vi "pruebausuario.vi"() -> ()   [LabVIEW 2018]
uses:
  Tabcontrol.ctl
panel:
  out "element":string
  out "Tab Control 2":enum32{"Login", "Usuarios", "Admin"}(tab)
  in  "Usuario 2":string
  in  "Contraseña 4":string
  in  "ingresar":bool
  in  "Contraseña U.I":string
  in  "Usuario a Ingresar":string
  in  "OK Button":bool
  in  "eliminar 2":bool
  out "array":string[][](array[string])
  out "result string":string
  out "Boolean":bool
  out "Contraseña 3":string
  in  "stop":bool
  out "appended path":path
  out "before substring":string
  out "match substring":string
  out "after substring":string
  out "text":string
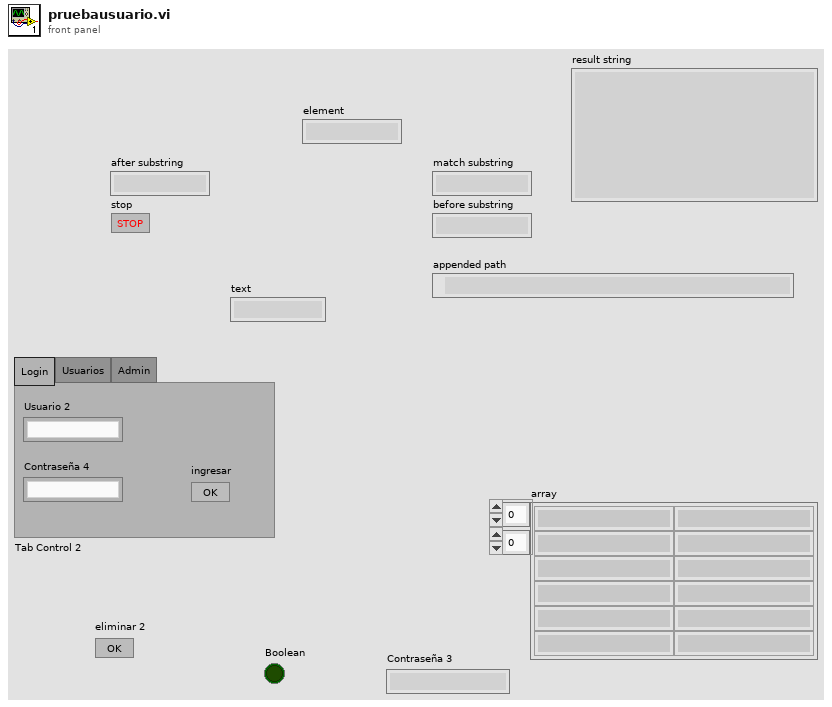
[diagram p1: front panel]
types:
  T1 = typedef "Tabcontrol.ctl" = enum16{"Login", "Usuarios", "Admin"}
  T2 = enum16{"open", "replace", "create", "open or create", "replace or create", "replace or create with confirmation"}
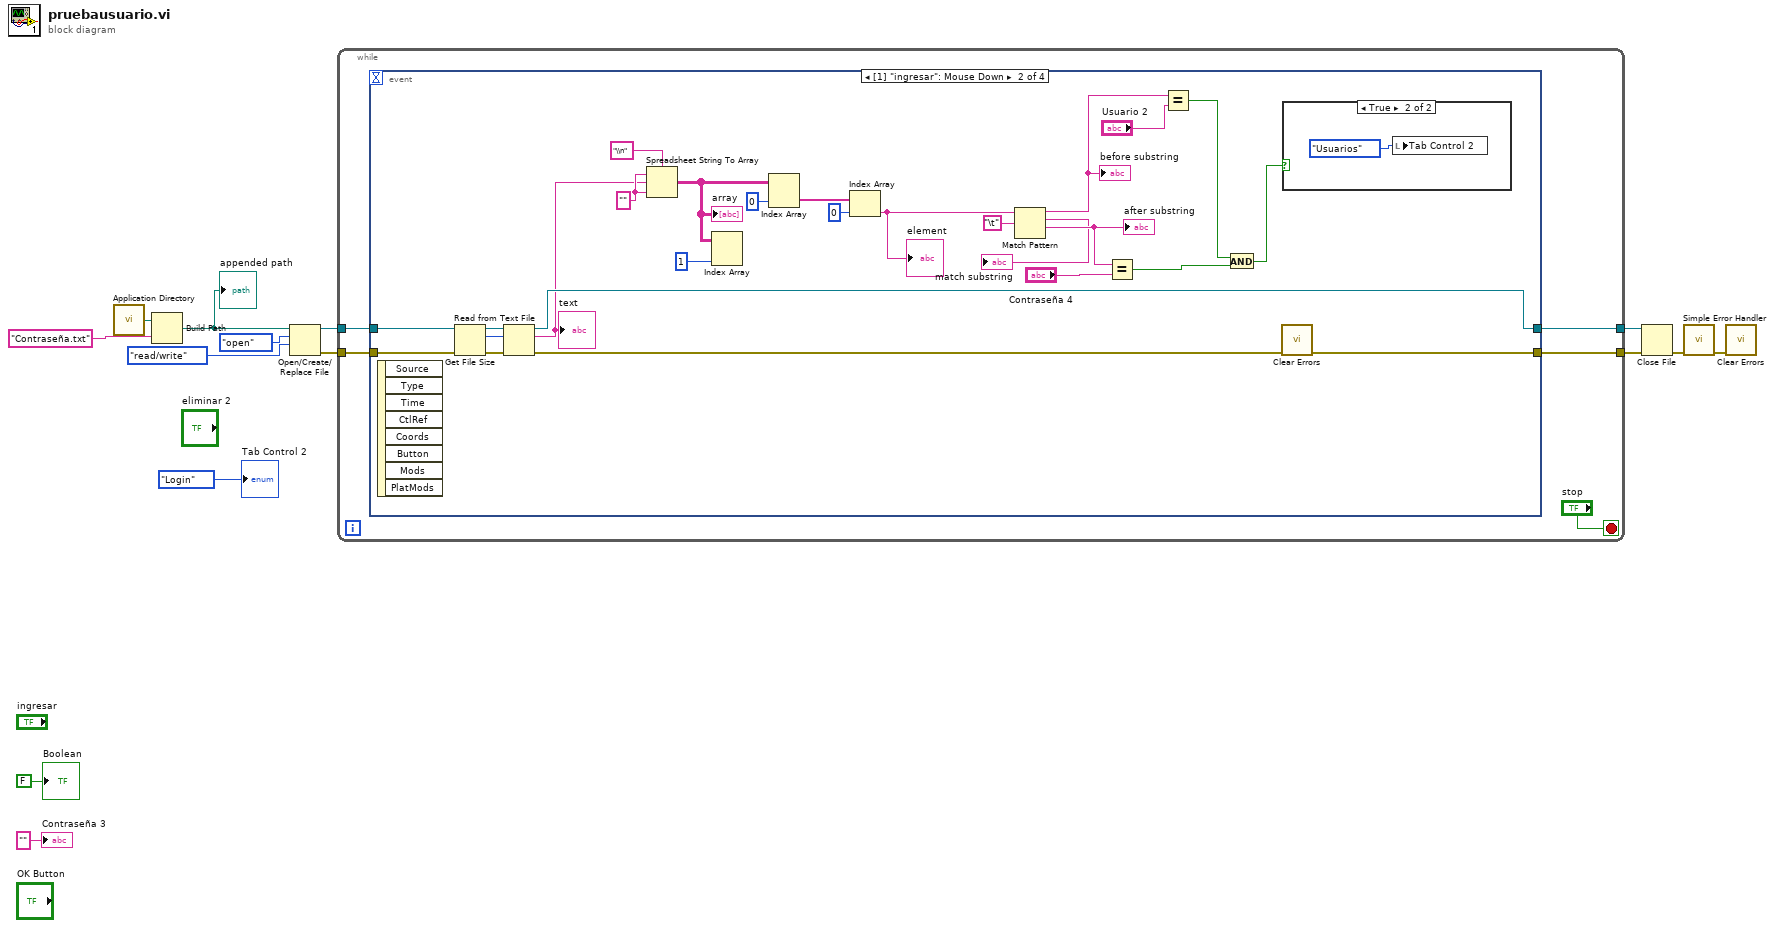
[diagram p0: block diagram]
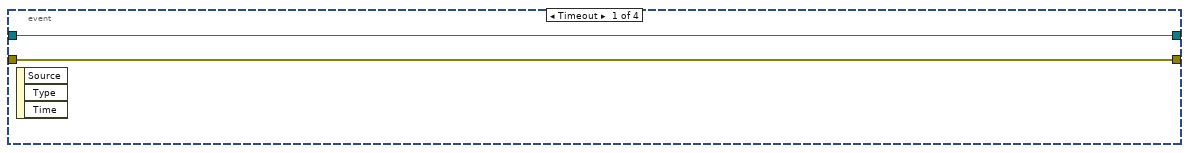
[diagram p2: hidden frame]
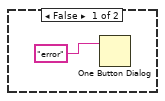
[diagram p3: hidden frame]
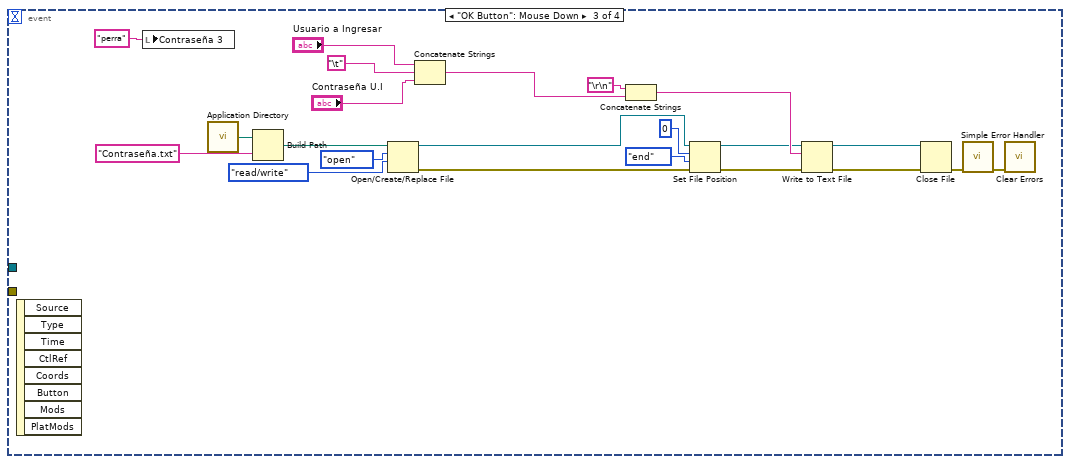
[diagram p4: hidden frame]
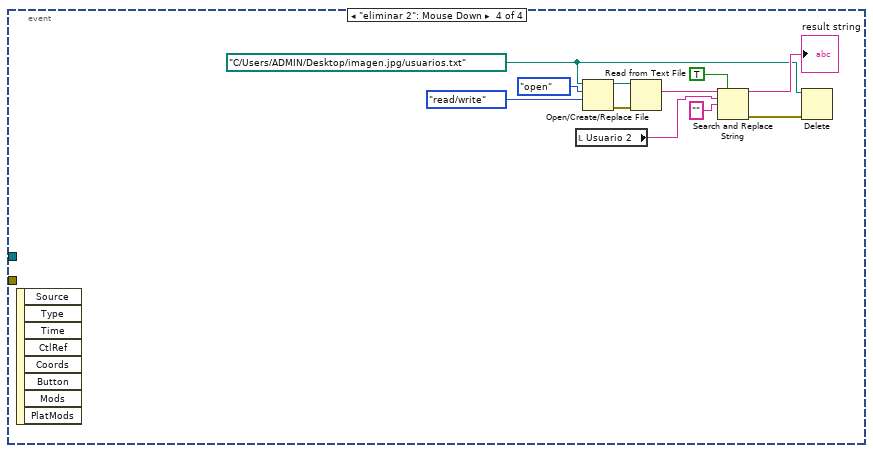
[diagram p5: hidden frame]
diagram:
  n1 = call <vilib>:"Application Directory.vi"() -> ("Application Directory"=w14:path)
  n2 = Build Path(base path=w14, name or relative path="Contraseña.txt") -> (appended path=w12:path)
  "appended path" <- w12
  n3 = Open/Create/Replace File(file path (use dialog)=w12, operation (0:open)=T2."open", access (0:read/write)=enum16{"read/write", "read-only", "write-only"}."read/write") -> (refnum out=w10:refnum<file>, error out=w11:errorcluster)  [unwired: 3 in, 1 out]
  n4 = while {
    tunnel: w11 -> [w19]
    tunnel: w10 -> [w18]
    tunnel: [w17] -> w9
    tunnel: [w16] -> w8
    stop <- "stop" stop-if-true
    n5 = event shown="[1] \"ingresar\": Mouse Down" {
      selector: _ -> [_ _ _ _]
      dyn-events: _ -> [_ _ _ _]
      timeout: _ -> [_ _ _ _]
      tunnel: w19 -> [w20 w37 _ _]
      tunnel: w18 -> [w21 w38 _ _]
      tunnel: [w20 w33 _ _] -> w17
      tunnel: [w21 w40 _ _] -> w16
      event Timeout {
        n6 = event-data() -> ()  [unwired: 1 in, 3 out]
      }
      event "ingresar": Mouse Down {
        w32 = "" ("format string")
        n7 = event-data() -> ()  [unwired: 1 in, 8 out]
        n8 = Get File Size(file=w38, error in=w37) -> (refnum out=w35:refnum<file>, size (in bytes)=w34:i64, 0:w36:errorcluster)
        n9 = Read from Text File(file (use dialog)=w35, count=w34, error in=w36) -> (refnum out=w40:refnum<file>, text=w31:string, error out=w41:errorcluster)  [unwired: 1 in, 1 out]
        "text" <- w31
        n10 = Spreadsheet String To Array(delimiter (Tab)="\\n", format string=w32, spreadsheet string=w31, array type (2D Dbl)=w32) -> (array=w28:string[][])
        "array" <- w28
        n11 = Index Array(array=w28, index (col)=1 ("index")) -> ()  [unwired: 1 in, 1 out]
        n12 = Index Array(array=w28, index (col)=0) -> (element=w27:string[])  [unwired: 1 in]
        n13 = Index Array(array=w27, index=0) -> (element=w23:string)
        "element" <- w23
        n14 = Match Pattern(string=w23, regular expression="\t") -> (before substring=w45:string, match substring=→"match substring":string, after substring=w47:string)  [unwired: 1 in, 1 out]
        "after substring" <- w47
        "before substring" <- w45
        n15 = Equal?(x=w47, y="Contraseña 4") -> (x = y?=w43:bool)
        n16 = Equal?(x=w45, y="Usuario 2") -> (x = y?=w44:bool)
        n17 = And(x=w44, y=w43) -> (x .and. y?=w42:bool)
        n18 = call <vilib>:"Clear Errors.vi"("error in (no error)"=w41) -> ("error out"=w33:errorcluster)  [unwired: 5 in, 1 out]
        n19 = case shown="True" w42 {
          frame False {
            n20 = One Button Dialog(message="error") -> ()  [unwired: 1 in, 1 out]
          }
          frame True {
            n21 = local write "Tab Control 2"(Tabcontrol."Usuarios") -> ()
          }
        }
      }
      event "OK Button": Mouse Down {
        n22 = event-data() -> ()  [unwired: 1 in, 8 out]
        n23 = local write "Contraseña 3"("perra" ("Contraseña 3")) -> ()
        n24 = call <vilib>:"Application Directory.vi"() -> ("Application Directory"=w70:path)
        n25 = Build Path(base path=w70, name or relative path="Contraseña.txt") -> (appended path=w69:path)
        n26 = Open/Create/Replace File(file path (use dialog)=w69, operation (0:open)=T2."open", access (0:read/write)=enum16{"read/write", "read-only", "write-only"}."read/write") -> (refnum out=w56:refnum<file>, error out=w55:errorcluster)  [unwired: 3 in, 1 out]
        n27 = Concatenate Strings "Concatenate Strings"("Usuario a Ingresar", "\t", "Contraseña U.I") -> (w60:string)
        n28 = Concatenate Strings "Concatenate Strings"("\r\n", w60) -> (w59:string)
        n29 = Set File Position(offset (in bytes) (0)=i64 0, refnum=w56, from (0:start)=enum16{"start", "end", "current"}."end", error in=w55) -> (refnum out=w54:refnum<file>, error out=w53:errorcluster)
        n30 = Write to Text File(file (use dialog)=w54, text=w59, error in=w53) -> (refnum out=w66:refnum<file>, error out=w65:errorcluster)  [unwired: 1 in, 1 out]
        n31 = Close File(refnum=w66, error in=w65) -> (error out=w67:errorcluster)  [unwired: 1 out]
        n32 = call <vilib>:"Simple Error Handler.vi"("error in (no error)"=w67) -> ("error out"=w68:errorcluster)  [unwired: 4 in, 4 out]
        n33 = call <vilib>:"Clear Errors.vi"("error in (no error)"=w68) -> ()  [unwired: 5 in, 2 out]
      }
      event "eliminar 2": Mouse Down {
        w74 = path "C:/Users/ADMIN/Desktop/imagen.jpg/usuarios.txt" ("path")
        n34 = event-data() -> ()  [unwired: 1 in, 8 out]
        n35 = local read "Usuario 2"() -> (w72:string)
        n36 = Open/Create/Replace File(file path (use dialog)=w74, operation (0:open)=T2."open", access (0:read/write)=enum16{"read/write", "read-only", "write-only"}."read/write") -> (refnum out=w79:refnum<file>, error out=w80:errorcluster)  [unwired: 3 in, 1 out]
        n37 = Read from Text File(file (use dialog)=w79, error in=w80) -> (text=w78:string)  [unwired: 2 in, 3 out]
        n38 = Search and Replace String(replace all?=TRUE ("replace all? (F)"), input string=w78, search string=w72, replace string="" ("replace string (\"\")")) -> (result string=→"result string":string, error out=w73:errorcluster)  [unwired: 4 in, 2 out]
        n39 = Delete(path (use dialog)=w74, error in=w73) -> ()  [unwired: 3 in, 3 out]
      }
    }
  }
  n40 = Close File(refnum=w8, error in=w9) -> (error out=w7:errorcluster)  [unwired: 1 out]
  n41 = call <vilib>:"Simple Error Handler.vi"("error in (no error)"=w7) -> ("error out"=w6:errorcluster)  [unwired: 4 in, 4 out]
  n42 = call <vilib>:"Clear Errors.vi"("error in (no error)"=w6) -> ()  [unwired: 5 in, 2 out]
  "Contraseña 3" <- "" ("Contraseña 3")
  "Boolean" <- FALSE ("Boolean")
  "Tab Control 2" <- Tabcontrol."Login"
